vi "Create Data Table By Name.vi"(8 "error in (no error)":errorcluster caption="错误输入（无错误）", 10 "tableName":string, 11 "DataTable 输入":refnum<class "DataTable.lvclass"> caption="DNL_LabVIEW Object in") -> (0 "error out":errorcluster caption="错误输出", 3 "DataTable 输出":refnum<class "DataTable.lvclass"> caption="DNL_LabVIEW Object out")   [LabVIEW 2012, in "Data Grid VIEW.lvlib" / "DataTable.lvclass"]
uses:
  DataTable.lvclass
  System.Data
  DataTable.lvclass/DataTable.ctl
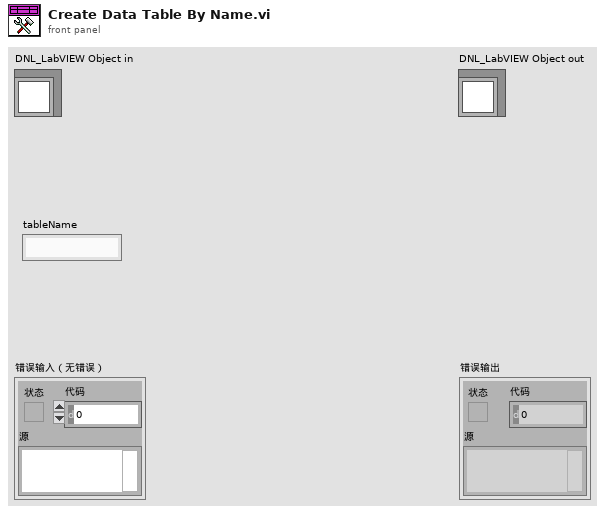
[diagram p1: front panel]
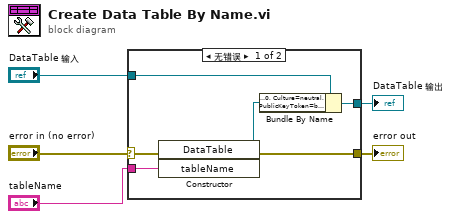
[diagram p0: block diagram]
diagram:
  n1 = case shown="无错误" "error in (no error)" {
    selector: "error in (no error)" -> [w8 w13]
    tunnel: [w7 w13] -> w4
    tunnel: [w9 w12] -> w2
    tunnel: "DataTable 输入" -> [w11 w12]
    tunnel: "tableName" -> [w6 _]
    frame No Error {
      n2 = constructor class="DataTable"(error in=w8, "tableName"=w6) -> (reference out=w10:refnum<k24>, error out=w7:errorcluster)  [unwired: 2 in, 2 out]
      n3 = Bundle By Name(cluster=w11, "DataTable"=w10) -> (w9:refnum<class "DataTable.lvclass">)
    }
    frame Error {
    }
  }
  "error out" <- w4
  "DataTable 输出" <- w2
